vi "Get Chassis and modules list.vi"(8 "error in":errorcluster caption="error in (no error)") -> (0 "error out":errorcluster, 1 "Chassis list":string[](array[string]), 2 "Modules Out":string[][](array[string]), 3 "Status Out":T1)   [LabVIEW 2011]
uses:
  Controls/HW Server Status.ctl
  Controls/ModuleCluster.ctl
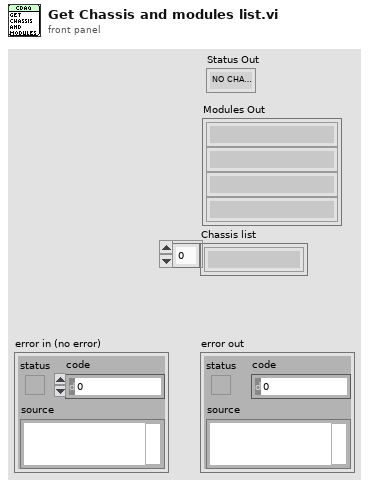
[diagram p1: front panel]
types:
  T1 = typedef "HW Server Status.ctl" = enum16{"NO CHASSIS", "NO MODULES", "OK"}
  T2 = typedef "ModuleCluster.ctl" = cluster{"Device Ref":refnum<k20>, "ProdName":string, "ConnLink":string, "Alias":string}
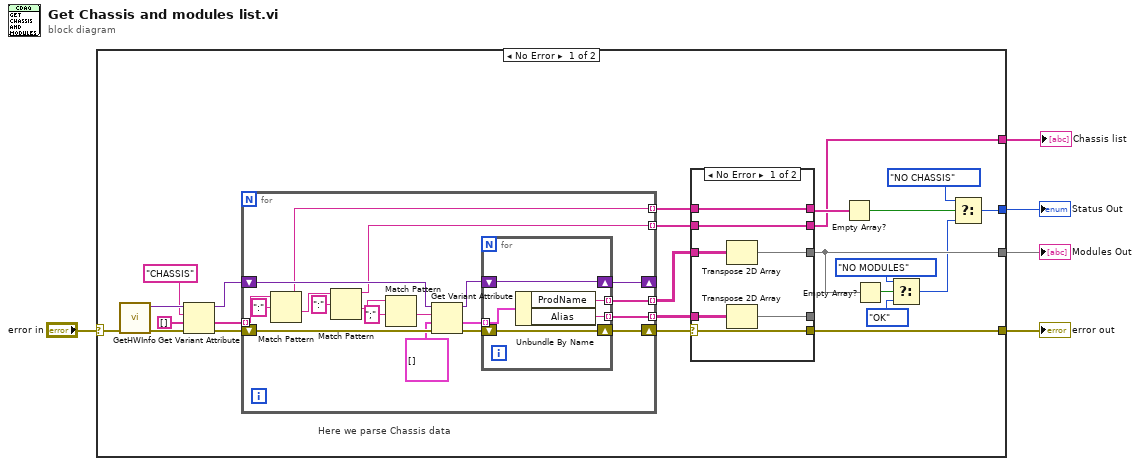
[diagram p0: block diagram]
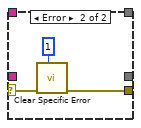
[diagram p2: hidden frame]
diagram:
  n1 = case shown="No Error" "error in" {
    selector: "error in" -> [w21 w64]
    tunnel: [w15 _] -> w5
    tunnel: [w16 w64] -> w4
    tunnel: [w8 _] -> w2
    tunnel: [w6 _] -> w1
    frame No Error {
      # "Here we parse Chassis data"
      n2 = call "GetHWInfo.vi"("error in"=w21) -> ("error out"=w29:errorcluster, "Refs Out"=w28:variant)  [unwired: 9 in]
      n3 = Get Variant Attribute(Variant=w28, name="CHASSIS", default value (empty Variant)=string[] [], error in=w29) -> (duplicate Variant=w23:variant, value=w24:string[], error out=w25:errorcluster)  [unwired: 1 out]
      n4 = for {
        shift-right: [w50] -> w20
        shift-left: w25 -> [w58]
        tunnel: w24 -> [w41] mode=indexing
        shift-right: [w52] -> _
        shift-left: w23 -> [w57]
        tunnel: [w51] -> w22 mode=indexing
        tunnel: [w49] -> w19 mode=indexing
        tunnel: [w44] -> w17 mode=indexing
        tunnel: [w40] -> w18 mode=indexing
        n5 = Match Pattern(string=w41, regular expression=":") -> (before substring=w40:string, after substring=w42:string)  [unwired: 1 in, 2 out]
        n6 = Match Pattern(string=w42, regular expression=":") -> (before substring=w49:string, after substring=w46:string)  [unwired: 1 in, 2 out]
        n7 = Match Pattern(string=w46, regular expression=";") -> (before substring=w45:string)  [unwired: 1 in, 3 out]
        n8 = Get Variant Attribute(Variant=w57, name=w45, default value (empty Variant)=T2[] [] ("appended array"), error in=w58) -> (duplicate Variant=w53:variant, value=w55:T2[], error out=w54:errorcluster)  [unwired: 1 out]
        n9 = for {
          tunnel: w55 -> [w62] mode=indexing
          shift-right: [w60] -> w50
          shift-left: w54 -> [w60]
          shift-right: [w63] -> w52
          shift-left: w53 -> [w63]
          tunnel: [w61] -> w51 mode=indexing
          tunnel: [w59] -> w44 mode=indexing
          n10 = Unbundle By Name(w62) -> ("ProdName"=w61:string, "Alias"=w59:string)
        }
      }
      n11 = case shown="No Error" w20 {
        selector: w20 -> [w33 w38]
        tunnel: w22 -> [w36 _]
        tunnel: [w35 _] -> w15
        tunnel: w19 -> [w34 _]
        tunnel: [w34 _] -> w6
        tunnel: [w33 w37] -> w16
        tunnel: w18 -> [w32 _]
        tunnel: [w32 _] -> w7
        tunnel: w17 -> [w31 _]
        tunnel: [w30 _] -> _
        frame No Error {
          n12 = Transpose 2D Array(2D array=w36) -> (transposed array=w35:string[][])
          n13 = Transpose 2D Array(2D array=w31) -> (transposed array=w30:string[][])
        }
        frame Error {
          n14 = call "Clear Specific Error.vi"("code"=1, "error in (no error)"=w38) -> ("error out"=w37:errorcluster)  [unwired: 9 in]
        }
      }
      n15 = Empty Array?(array=w7) -> (empty?=w13:bool)
      n16 = Empty Array?(array=w15) -> (empty?=w14:bool)
      n17 = Select(t=HW_Server_Status."NO MODULES", s=w14, f=HW_Server_Status."OK") -> (s? t:f=w10:T1)
      n18 = Select(t=HW_Server_Status."NO CHASSIS", s=w13, f=w10) -> (s? t:f=w8:T1)
    }
    frame Error {
    }
  }
  "Modules Out" <- w5
  "error out" <- w4
  "Status Out" <- w2
  "Chassis list" <- w1
